vi "Main.vi"(11 "Module Admin":refnum<class "Delacor_lib_QMH_Cloneable Module Admin.lvclass">) -> ()   [LabVIEW 2018, in "CE14 eMIC module.lvlib"]
doc: "This template is based off of the Queued Message Handler design pattern and the Queued Message Handler project template that ships with LabVIEW.\n\nThe main difference is that the queue is private to this module and communication between modules is performed via Broadcast and Request events.\n\nRequest events are wrapped in public API methods and are handled in the Event Handling Loop (EHL) of this VI. Any module can register for Broadcast events sent by this module. The EHL generates messages based on user interface actions.\n\nThe Message Handling Loop (MHL) processes messages generated by the EHL, or by other messages. The messages are string values, so new messages can be added easily to the Message Cases case structure in the MHL. Each message cluster can also provide an optional value for Message Data, which is a variant that can be converted to whatever message-specific data is required.\n_____\nBased on DQMH Project Template 6.0.0.91."
uses:
  CE14 eMIC module.lvlib
  <vilib>/Delacor/Delacor QMH/Libraries/Cloneable Module Admin_class/Delacor_lib_QMH_Cloneable Module Admin.lvclass
  C:/Program Files (x86)/National Instruments/LabVIEW 2018/vi.lib/Delacor/Delacor QMH/Libraries/Module Admin_class/Delacor_lib_QMH_Module Admin.lvclass
  Module Data--cluster.ctl
  Do Something Argument--cluster.ctl
  <vilib>/Delacor/Delacor QMH/Libraries/Cloneable Module Admin_class/Delacor_lib_QMH_Cloneable Module Admin.lvclass/Delacor_lib_QMH_Cloneable Module Admin.ctl
  <vilib>/Delacor/Delacor QMH/Libraries/Message Queue_class/Delacor_lib_QMH_Message Queue.lvclass/Delacor_lib_QMH_Message Queue.ctl
  Do Something Else Argument--cluster.ctl
  Do Something Else and Wait for Reply Argument--cluster.ctl
  Do Something Else and Wait (Reply Payload)--cluster.ctl
  Stop Argument--cluster.ctl
  <vilib>/Delacor/Delacor QMH/Libraries/Module Admin_class/Delacor_lib_QMH_Module Admin.lvclass/Delacor_lib_QMH_Module Admin.ctl
  Open&shakehand eMICs Argument--cluster.ctl
  Open&shakehand eMICs (Reply Payload)--cluster.ctl
  <vilib>/Utility/miscctls.llb/LVPointTypeDef.ctl
  <vilib>/Delacor/Delacor QMH/Libraries/Message Queue_class/Delacor_lib_QMH_Enqueue Message (Single).vi
  <vilib>/Delacor/Delacor QMH/Libraries/Cloneable Module Admin_class/Delacor_lib_QMH_Get Module ID.vi
  <vilib>/Delacor/Delacor QMH/Libraries/Module Admin_class/Delacor_lib_QMH_Get External Launch.vi
  <vilib>/Utility/error.llb/Error Cluster From Error Code.vi
  <vilib>/ErrorRing/Error Ring.xnode
  <vilib>/Delacor/Delacor QMH/Libraries/Message Queue_class/Delacor_lib_QMH_Message Queue.lvclass
  Instrument Drivers/LVdriver_CE14(eMIC)/CE14_eMIC.lvlib
panel:
  out "error out":errorcluster
  out "X":dbl
  out "Status":string
  in  "Simulate EHL Error":bool
  in  "Simulate MHL Error":bool
  in  "Do Something Else <Replace Me>":bool
  in  "Do Something <Replace Me>":bool
  # "These controls have associated \"Value Changed\" events configured in the Event Structure on the diagram.\n\nReplace them (and reconfigure the Event Structure) with the controls you need for your application. \n\nOther QMH Modules communicate with this Module via its Public API (wrappers for its Request Events).\n\nThis Module communicates with other Modules via its Broadcast Events.\nAny module that wants to get these messages, just registers for this module's Broadcast events."
  # "This template is for the Delacor Modified Queued Message Handler design pattern.\n\nSee the block diagram for more information on how to use this template."
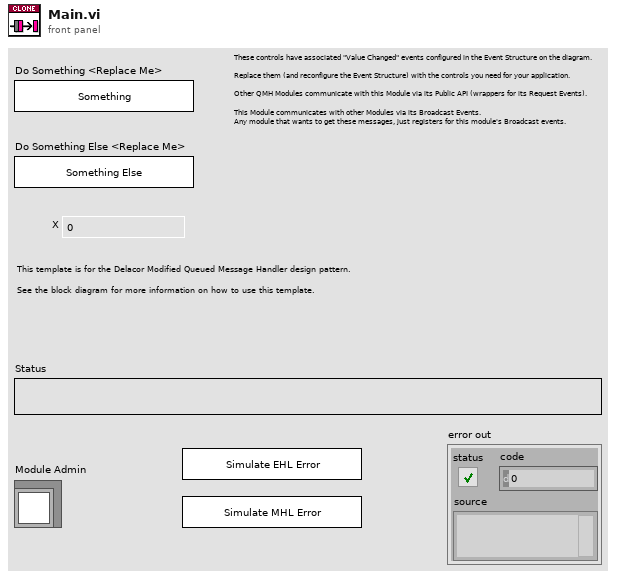
[diagram p1: front panel]
types:
  T1 = typedef "CE14 eMIC module.lvlib/Request Events--cluster.ctl" = cluster{"Stop Module":refnum<user-event>, "Do Something":refnum<user-event>, "Do Something Else":refnum<user-event>, "Do Something Else and Wait for Reply":refnum<user-event>, "Show Panel":refnum<user-event>, "Hide Panel":refnum<user-event>, "Show Diagram":refnum<user-event>, "Get Module Execution Status":refnum<user-event>, "Open&shakehand eMICs":refnum<user-event>}
  T2 = typedef "CE14 eMIC module.lvlib/Module Data--cluster.ctl" = cluster{"Status":string, "VISA resource name":refnum<visa-resource-name>}
  T3 = typedef "CE14 eMIC module.lvlib/Do Something Argument--cluster.ctl" = cluster{"Module ID":i32, "Do Something Msg":string}
  T4 = typedef "CE14 eMIC module.lvlib/Do Something Else Argument--cluster.ctl" = cluster{"Module ID":i32, "Do Something Else Msg":string, "X":dbl}
  T5 = typedef "CE14 eMIC module.lvlib/Do Something Else and Wait for Reply Argument--cluster.ctl" = cluster{"Module ID":i32, "Do Something Else Msg":string, "X":dbl, "Wait Notifier":refnum<notifier>, "wait for reply":bool}
  T6 = enum32{"invalid lock state", "Not Locked", "Locked (No Password)", "Password-protected"}
  T7 = typedef "CE14 eMIC module.lvlib/Stop Argument--cluster.ctl" = cluster{"Module ID":i32, "Origin":string, "Exit via Stop Module Req?":bool, "Wait for Module to stop?":bool}
  T8 = typedef "CE14 eMIC module.lvlib/Open&shakehand eMICs Argument--cluster.ctl" = cluster{"Module ID":i32, "VISA resource name":refnum<visa-resource-name>, "Wait Notifier":refnum<notifier>, "wait for reply":bool}
  T9 = typedef "LVPointTypeDef.ctl" = cluster{"Horizontal":i16, "Vertical":i16}
  T10 = enum32{"Invalid", "Standard", "Closed", "Hidden", "Minimized", "Maximized"}
  T11 = typedef "CE14 eMIC module.lvlib/Do Something Else and Wait (Reply Payload)--cluster.ctl" = cluster{"Value":dbl, "error":errorcluster}
  T12 = typedef "CE14 eMIC module.lvlib/Open&shakehand eMICs (Reply Payload)--cluster.ctl" = cluster{"success":bool, "Open&shakehand eMICs_error":errorcluster}
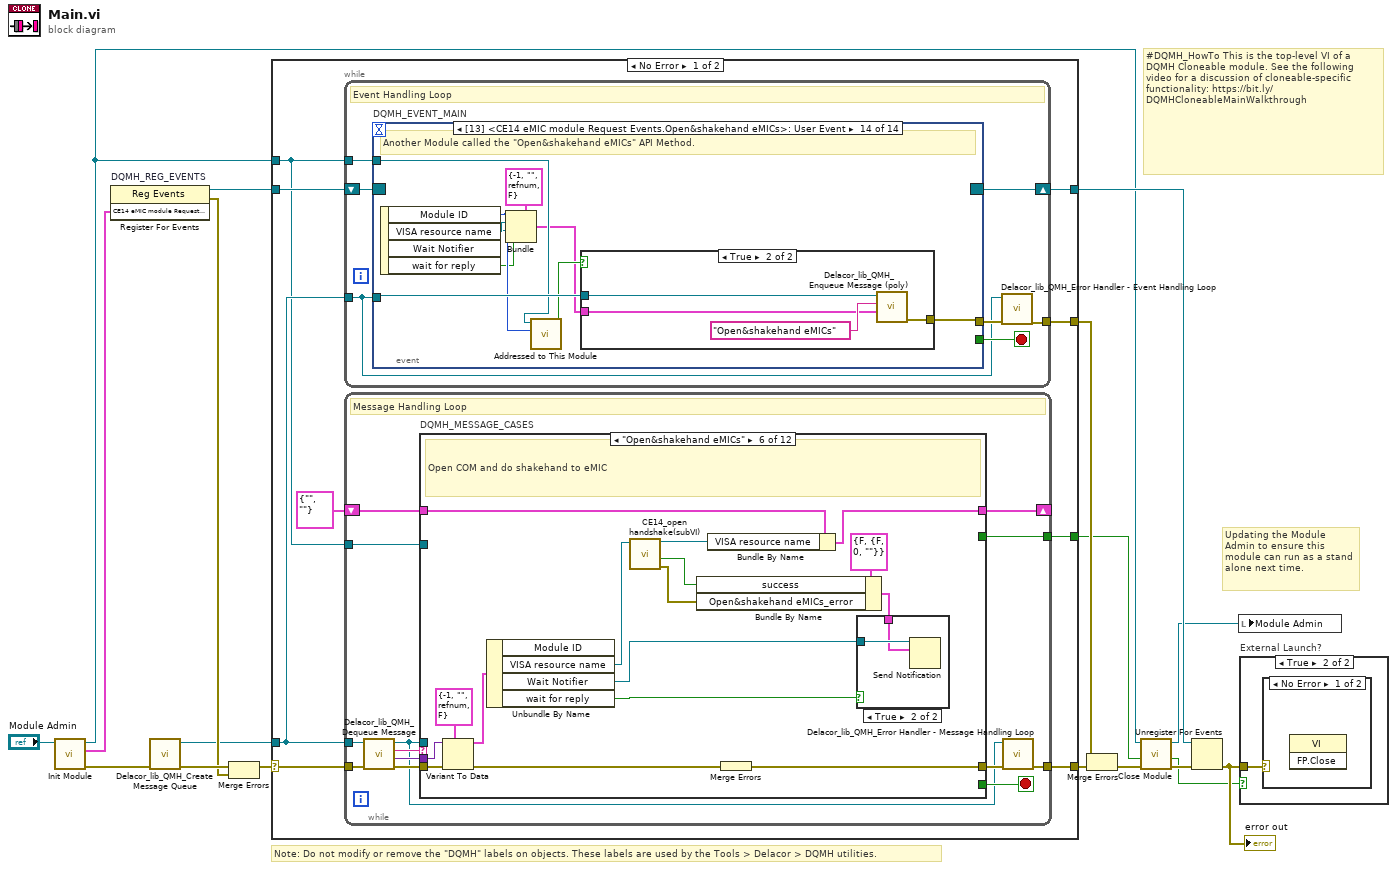
[diagram p0: block diagram]
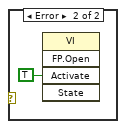
[diagram p3: hidden frame]
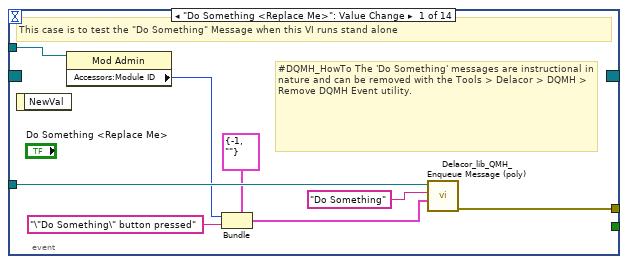
[diagram p4: hidden frame]
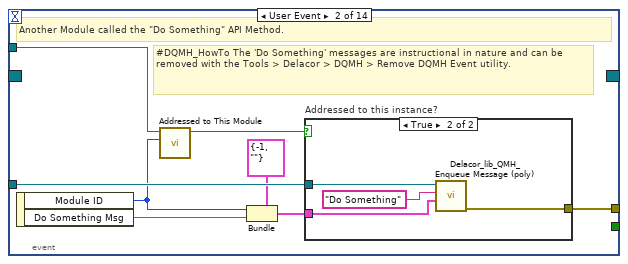
[diagram p5: hidden frame]
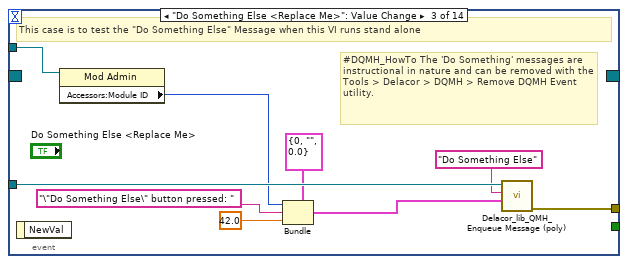
[diagram p7: hidden frame]
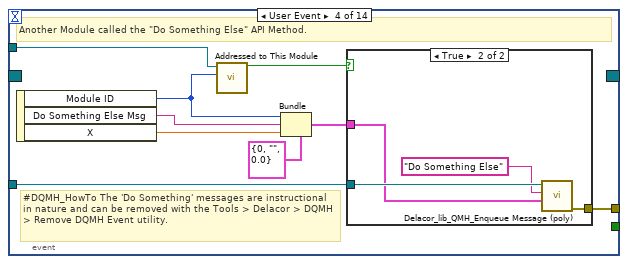
[diagram p8: hidden frame]
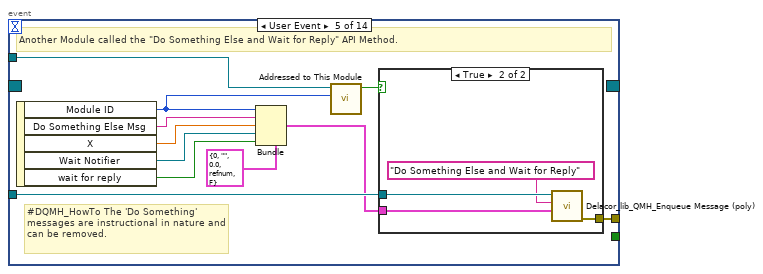
[diagram p10: hidden frame]
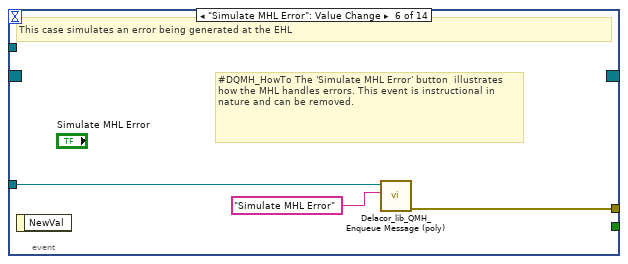
[diagram p12: hidden frame]
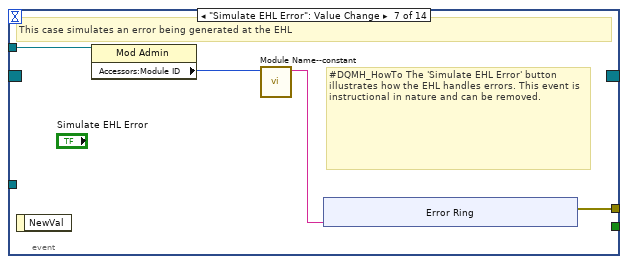
[diagram p13: hidden frame]
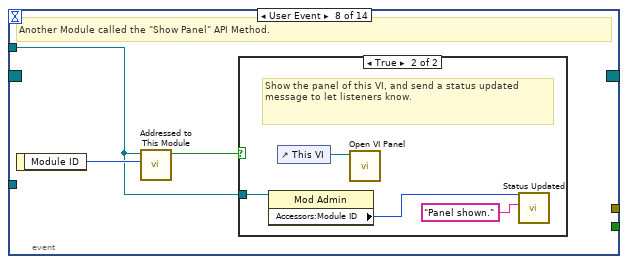
[diagram p14: hidden frame]
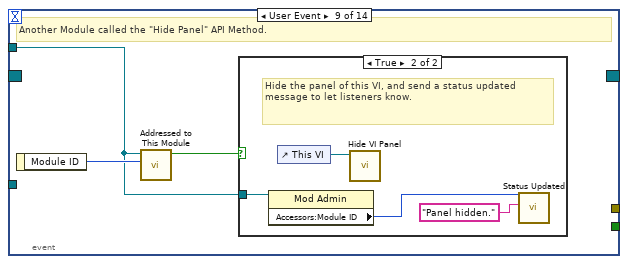
[diagram p16: hidden frame]
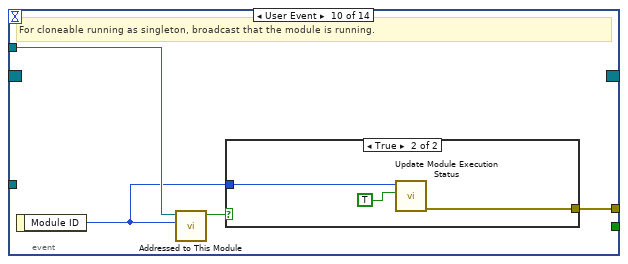
[diagram p18: hidden frame]
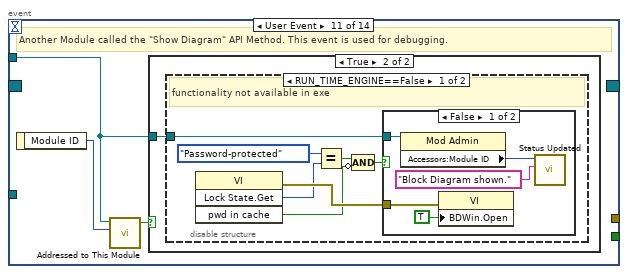
[diagram p20: hidden frame]
diagram:
  # "#DQMH_HowTo This is the top-level VI of a DQMH Cloneable module. See the following video for a discussion of cloneable-specific functionality: https://bit.ly/DQMHCloneableMainWalkthrough"
  # "Note: Do not modify or remove the \"DQMH\" labels on objects. These labels are used by the Tools > Delacor > DQMH utilities."
  # "Updating the Module Admin to ensure this module can run as a stand alone next time."
  n1 = call "Init Module.vi"("Cloneable Module Admin in"="Module Admin") -> ("error out"=w15:errorcluster, "CE14 eMIC module Request Events"=w7:T1, "Cloneable Module Admin out"=w4:refnum<class "Delacor_lib_QMH_Cloneable Module Admin.lvclass">)  [unwired: 8 in]
  n2 = register-events "DQMH_REG_EVENTS"(w7) -> (reference out=w8:refnum<event-registration>, error out=w10:errorcluster)  [unwired: 2 in]
  n3 = call <vilib>:"Delacor_lib_QMH_Create Message Queue.vi"("error in"=w15) -> ("error out"=w12:errorcluster, "Message Queue"=w6:refnum<class "Delacor_lib_QMH_Message Queue.lvclass">)  [unwired: 9 in]
  n4 = Merge Errors(w12, w10) -> (w11:errorcluster)
  n5 = case shown="No Error" w11 {
    selector: w11 -> [w25 w366]
    tunnel: [w27 w365] -> w16
    tunnel: [w24 w373] -> w9
    tunnel: w8 -> [w22 w373]
    tunnel: w6 -> [w21 w364]
    tunnel: [w26 _] -> w17
    tunnel: w4 -> [w20 w369]
    tunnel: [w19 _] -> w2
    frame No Error {
      n6 = while {
        tunnel: w21 -> [w28]
        shift-right: [w31] -> w24
        shift-left: w22 -> [w32]
        tunnel: [w33] -> w26
        tunnel: w20 -> [w29]
        stop <- w30 stop-if-true
        # "Event Handling Loop"
        n7 = event "DQMH_EVENT_MAIN" shown="[13] <CE14 eMIC module Request Events.Open&shakehand eMICs>: User Event" {
          selector: w32 -> [_ _ _ _ _ _ _ _ _ _ _ _ _ _]
          dyn-events: [_ _ _ _ _ _ _ _ _ _ _ _ _ _] -> w31
          timeout: _ -> [_ _ _ _ _ _ _ _ _ _ _ _ _ _]
          tunnel: [_ _ _ _ _ _ _ _ _ _ _ w146 _ _] -> w30
          tunnel: w28 -> [w41 w49 w62 w71 w86 w93 _ _ _ _ _ w149 w165 w183]
          tunnel: [w42 w50 w63 w72 w87 w94 w98 _ _ w123 _ w150 w168 w174] -> w34
          tunnel: w29 -> [w37 w47 w56 w69 w84 _ w97 w106 w113 w121 w127 w148 w166 w181]
          event "Do Something <Replace Me>": Value Change {
            # "#DQMH_HowTo The 'Do Something' messages are instructional in nature and can be removed with the Tools > Delacor > DQMH > Remove DQMH Event utility."
            # "This case is to test the \"Do Something\" Message when this VI runs stand alone"
            n8 = event-data() -> ()  [unwired: 1 in, 1 out]
            n9 = property class="Mod Admin"(reference=w37) -> ("Accessors:Module ID"=w36:i32)  [unwired: 1 in, 2 out]
            n10 = Bundle(cluster=T3 {"Module ID"=-1, "Do Something Msg"=""} ("Do Something Argument"), "Module ID"=w36, "Do Something Msg"="\"Do Something\" button pressed" ("\"Do Something\" button pressed")) -> (w39:T3)
            n11 = call-poly <vilib>:"Delacor_lib_QMH_Enqueue Message (poly).vi"("Message Data"=w39, "Message"="Do Something", "Message Queue in"=w41) -> ("error out"=w42:errorcluster)  [unwired: 7 in, 1 out]
          }
          event User Event {
            # "#DQMH_HowTo The 'Do Something' messages are instructional in nature and can be removed with the Tools > Delacor > DQMH > Remove DQMH Event utility."
            # "Another Module called the \"Do Something\" API Method."
            n12 = event-data() -> ("Module ID"=w44:i32, "Do Something Msg"=w43:string)  [unwired: 1 in]
            n13 = call "Addressed to This Module.vi"("Module ID from Argument"=w44, "Module Admin"=w47) -> ("Addressed to this instance?"=w48:bool)  [unwired: 8 in, 1 out]
            n14 = Bundle(cluster=T3 {"Module ID"=-1, "Do Something Msg"=""} ("Do Something Argument"), "Module ID"=w44, "Do Something Msg"=w43) -> (w46:T3)
            n15 = case "Addressed to this instance?" shown="True" w48 {
              tunnel: w49 -> [_ w53]
              tunnel: [_ w54] -> w50
              tunnel: w46 -> [_ w51]
              frame False {
                # "Do nothing"
              }
              frame True {
                n16 = call-poly <vilib>:"Delacor_lib_QMH_Enqueue Message (poly).vi"("Message Data"=w51, "Message"="Do Something", "Message Queue in"=w53) -> ("error out"=w54:errorcluster)  [unwired: 7 in, 1 out]
              }
            }
          }
          event "Do Something Else <Replace Me>": Value Change {
            # "#DQMH_HowTo The 'Do Something' messages are instructional in nature and can be removed with the Tools > Delacor > DQMH > Remove DQMH Event utility."
            # "This case is to test the \"Do Something Else\" Message when this VI runs stand alone"
            n17 = event-data() -> ()  [unwired: 1 in, 1 out]
            n18 = property class="Mod Admin"(reference=w56) -> ("Accessors:Module ID"=w55:i32)  [unwired: 1 in, 2 out]
            n19 = Bundle(cluster=T4 {"Module ID"=0, "Do Something Else Msg"="", "X"=0.0} ("Do Something Else Argument"), "Module ID"=w55, "Do Something Else Msg"="\"Do Something Else\" button pressed: " ("\"Do Something Else\" button pressed"), "X"=42.0) -> (w59:T4)
            n20 = call-poly <vilib>:"Delacor_lib_QMH_Enqueue Message (poly).vi"("Message Data"=w59, "Message"="Do Something Else", "Message Queue in"=w62) -> ("error out"=w63:errorcluster)  [unwired: 7 in, 1 out]
          }
          event User Event {
            # "#DQMH_HowTo The 'Do Something' messages are instructional in nature and can be removed with the Tools > Delacor > DQMH > Remove DQMH Event utility."
            # "Another Module called the \"Do Something Else\" API Method."
            n21 = event-data() -> ("Module ID"=w64:i32, "Do Something Else Msg"=w65:string, "X"=w67:dbl)  [unwired: 1 in]
            n22 = call "Addressed to This Module.vi"("Module ID from Argument"=w64, "Module Admin"=w69) -> ("Addressed to this instance?"=w70:bool)  [unwired: 8 in, 1 out]
            n23 = Bundle(cluster=T4 {"Module ID"=0, "Do Something Else Msg"="", "X"=0.0} ("Do Something Else Argument"), "Module ID"=w64, "Do Something Else Msg"=w65, "X"=w67) -> (w66:T4)
            n24 = case shown="True" w70 {
              tunnel: w71 -> [_ w75]
              tunnel: [_ w76] -> w72
              tunnel: w66 -> [_ w73]
              frame False {
              }
              frame True {
                n25 = call-poly <vilib>:"Delacor_lib_QMH_Enqueue Message (poly).vi"("Message Data"=w73, "Message"="Do Something Else", "Message Queue in"=w75) -> ("error out"=w76:errorcluster)  [unwired: 7 in, 1 out]
              }
            }
          }
          event User Event {
            # "#DQMH_HowTo The 'Do Something' messages are instructional in nature and can be removed."
            # "Another Module called the \"Do Something Else and Wait for Reply\" API Method."
            n26 = event-data() -> ("Module ID"=w82:i32, "Do Something Else Msg"=w80:string, "X"=w79:dbl, "Wait Notifier"=w78:refnum<notifier>, "wait for reply"=w77:bool)  [unwired: 1 in]
            n27 = Bundle(cluster=T5 {"Module ID"=0, "Do Something Else Msg"="", "X"=0.0, "Wait Notifier"=refnum, "wait for reply"=FALSE} ("Do Something Else and Wait for Reply Argument"), "Module ID"=w82, "Do Something Else Msg"=w80, "X"=w79, "Wait Notifier"=w78, "wait for reply"=w77) -> (w81:T5)
            n28 = call "Addressed to This Module.vi"("Module ID from Argument"=w82, "Module Admin"=w84) -> ("Addressed to this instance?"=w85:bool)  [unwired: 8 in, 1 out]
            n29 = case shown="True" w85 {
              tunnel: [_ w91] -> w87
              tunnel: w86 -> [_ w90]
              tunnel: w81 -> [_ w88]
              frame False {
              }
              frame True {
                n30 = call-poly <vilib>:"Delacor_lib_QMH_Enqueue Message (poly).vi"("Message Data"=w88, "Message"="Do Something Else and Wait for Reply", "Message Queue in"=w90) -> ("error out"=w91:errorcluster)  [unwired: 7 in, 1 out]
              }
            }
          }
          event "Simulate MHL Error": Value Change {
            # "#DQMH_HowTo The 'Simulate MHL Error' button  illustrates how the MHL handles errors. This event is instructional in nature and can be removed."
            # "This case simulates an error being generated at the EHL"
            n31 = event-data() -> ()  [unwired: 1 in, 1 out]
            n32 = call-poly <vilib>:"Delacor_lib_QMH_Enqueue Message (poly).vi"("Message"="Simulate MHL Error", "Message Queue in"=w93) -> ("error out"=w94:errorcluster)  [unwired: 8 in, 1 out]
          }
          event "Simulate EHL Error": Value Change {
            # "#DQMH_HowTo The 'Simulate EHL Error' button  illustrates how the EHL handles errors. This event is instructional in nature and can be removed."
            # "This case simulates an error being generated at the EHL"
            n33 = event-data() -> ()  [unwired: 1 in, 1 out]
            n34 = property class="Mod Admin"(reference=w97) -> ("Accessors:Module ID"=w96:i32)  [unwired: 1 in, 2 out]
            n35 = call "Module Name--constant.vi"("Module ID"=w96) -> ("Module Name"=w95:string)  [unwired: 10 in]
            n36 = xnode "Error Ring"("parameter 0"=w95) -> ("error out"=w98:errorcluster)
          }
          event User Event {
            # "Another Module called the \"Show Panel\" API Method."
            n37 = event-data() -> ("Module ID"=w107:i32)  [unwired: 1 in]
            n38 = call "Addressed to This Module.vi"("Module ID from Argument"=w107, "Module Admin"=w106) -> ("Addressed to this instance?"=w108:bool)  [unwired: 8 in, 1 out]
            n39 = case shown="True" w108 {
              tunnel: w106 -> [_ w110]
              frame False {
              }
              frame True {
                # "Show the panel of this VI, and send a status updated message to let listeners know."
                n40 = property class="Mod Admin"(reference=w110) -> ("Accessors:Module ID"=w109:i32)  [unwired: 1 in, 2 out]
                n41 = control-ref of="This VI"() -> (w112:refnum<vi>)
                n42 = call "Open VI Panel.vi"("VI"=w112) -> ()  [unwired: 10 in, 1 out]
                n43 = call "Status Updated.vi"("Status"="Panel shown." ("format string"), "Module ID"=w109) -> ()  [unwired: 9 in, 1 out]
              }
            }
          }
          event User Event {
            # "Another Module called the \"Hide Panel\" API Method."
            n44 = event-data() -> ("Module ID"=w114:i32)  [unwired: 1 in]
            n45 = call "Addressed to This Module.vi"("Module ID from Argument"=w114, "Module Admin"=w113) -> ("Addressed to this instance?"=w115:bool)  [unwired: 8 in, 1 out]
            n46 = case shown="True" w115 {
              tunnel: w113 -> [_ w117]
              frame False {
              }
              frame True {
                # "Hide the panel of this VI, and send a status updated message to let listeners know."
                n47 = property class="Mod Admin"(reference=w117) -> ("Accessors:Module ID"=w116:i32)  [unwired: 1 in, 2 out]
                n48 = control-ref of="This VI"() -> (w119:refnum<vi>)
                n49 = call "Hide VI Panel.vi"("VI"=w119) -> ()  [unwired: 10 in, 1 out]
                n50 = call "Status Updated.vi"("Status"="Panel hidden." ("format string"), "Module ID"=w116) -> ()  [unwired: 9 in, 1 out]
              }
            }
          }
          event User Event {
            # "For cloneable running as singleton, broadcast that the module is running."
            n51 = event-data() -> ("Module ID"=w120:i32)  [unwired: 1 in]
            n52 = call "Addressed to This Module.vi"("Module ID from Argument"=w120, "Module Admin"=w121) -> ("Addressed to this instance?"=w122:bool)  [unwired: 8 in, 1 out]
            n53 = case shown="True" w122 {
              tunnel: [_ w126] -> w123
              tunnel: w120 -> [_ w125]
              frame False {
              }
              frame True {
                n54 = call "Update Module Execution Status.vi"("Running?"=TRUE, "Module ID"=w125) -> ("error out"=w126:errorcluster)  [unwired: 9 in]
              }
            }
          }
          event User Event {
            # "Another Module called the \"Show Diagram\" API Method. This event is used for debugging."
            n55 = event-data() -> ("Module ID"=w128:i32)  [unwired: 1 in]
            n56 = call "Addressed to This Module.vi"("Module ID from Argument"=w128, "Module Admin"=w127) -> ("Addressed to this instance?"=w129:bool)  [unwired: 8 in, 1 out]
            n57 = case shown="True" w129 {
              tunnel: w127 -> [_ w130]
              frame False {
              }
              frame True {
                n58 = disable-structure shown="RUN_TIME_ENGINE==False" {
                  disable-tunnel: w130 -> [w131 _]
                  frame condition #0 (active) {
                    # "functionality not available in exe"
                    n59 = invoke class="VI" method="Lock State.Get"() -> (error out=w137:errorcluster, "Get Lock State"=w136:T6, "pwd in cache"=w133:bool)  [unwired: 4 in, 1 out]
                    n60 = Equal?(x=T6."Password-protected", y=w136) -> (x = y?=w134:bool)
                    n61 = Compound Arithmetic op=AND(w134, invert w133) -> (w132:bool)
                    n62 = case shown="False" w132 {
                      tunnel: w137 -> [w142 _]
                      tunnel: w131 -> [w139 _]
                      frame False {
                        n63 = property class="Mod Admin"(reference=w139) -> ("Accessors:Module ID"=w138:i32)  [unwired: 1 in, 2 out]
                        n64 = property class="VI"(error in=w142, "BDWin.Open"=TRUE ("Block Diagram Window:Open")) -> ()  [unwired: 1 in, 2 out]
                        n65 = call "Status Updated.vi"("Status"="Block Diagram shown." ("format string"), "Module ID"=w138) -> ()  [unwired: 9 in, 1 out]
                      }
                      frame True {
                        # "Password-protected VI, and the password is not in the cache. Do not show the diagram."
                      }
                    }
                  }
                  frame condition #1 {
                  }
                }
              }
            }
          }
          event User Event {
            # "Another Module called the \"Stop Module\" API Method  or the Message Handling Loop below."
            n66 = event-data() -> ("Module ID"=w144:i32, "Wait for Module to stop?"=w145:bool, "Origin"=w143:string)  [unwired: 1 in]
            n67 = call "Addressed to This Module.vi"("Module ID from Argument"=w144, "Module Admin"=w148) -> ("Addressed to this instance?"=w147:bool)  [unwired: 8 in, 1 out]
            n68 = case shown="True" w147 {
              tunnel: [_ w162] -> w150
              tunnel: w149 -> [_ w158]
              tunnel: [_ TRUE] -> w146
              tunnel: w145 -> [_ w153]
              tunnel: w144 -> [_ w155]
              tunnel: w143 -> [_ w151]
              frame False {
              }
              frame True {
                # "The event can get fired from the Exit message. The queue gets destroyed there. In this case, the Enqueue VI will return error 1. It is safe to ignore, because the module is already exiting."
                n69 = local write "Status"(w151) -> ()
                n70 = Bundle By Name(cluster=T7 {"Module ID"=-1, "Origin"="", "Exit via Stop Module Req?"=FALSE, "Wait for Module to stop?"=FALSE} ("Stop Argument"), "Module ID"=w155, "Exit via Stop Module Req?"=TRUE, "Wait for Module to stop?"=w153) -> (w152:T7)
                n71 = call-poly <vilib>:"Delacor_lib_QMH_Enqueue Message (poly).vi"("Priority Message? (F)"=TRUE, "Message Data"=w152, "Message"="Exit", "Message Queue in"=w158) -> ("error out"=w163:errorcluster)  [unwired: 6 in, 1 out]
                n72 = call <vilib>:"Clear Errors.vi"("error in (no error)"=w163, "specific error code to clear (0: all)"=1) -> ("error out"=w162:errorcluster)  [unwired: 4 in, 1 out]
              }
            }
          }
          event Panel Close? {
            w167 = TRUE  # Discard the event, the MHL is responsible for closing and stopping this VI.
            # "Hide the panel or send the 'Exit' message if the user clicks the 'X' on the module main VI panel."
            n73 = event-data() -> ()  [unwired: 1 in, 1 out]
            n74 = property class="Mod Admin"(reference=w166) -> ("Accessors:External Launch"=w164:bool)  [unwired: 1 in, 2 out]
            n75 = case shown="True" w164 {
              tunnel: w165 -> [_ w172]
              tunnel: [_ w173] -> w168
              frame True {
                # "If externally launched, clicking the 'X' hides the panel, but doesn't close it."
                n76 = control-ref of="This VI"() -> (w169:refnum<vi>)
                n77 = call "Hide VI Panel.vi"("VI"=w169) -> ()  [unwired: 10 in, 1 out]
              }
              frame False {
                # "If run as a stand-alone VI, clicking the panel 'X' stops the VI."
                n78 = call-poly <vilib>:"Delacor_lib_QMH_Enqueue Message (poly).vi"("Priority Message? (F)"=TRUE, "Message"="Exit", "Message Queue in"=w172) -> ("error out"=w173:errorcluster)  [unwired: 7 in, 1 out]
              }
            }
            n79 = event-data("Discard?"=w167) -> ()  [unwired: 1 in, 1 out]
          }
          event User Event {
            # "Another Module called the \"Open&shakehand eMICs\" API Method."
            n80 = event-data() -> ("Module ID"=w178:i32, "VISA resource name"=w177:refnum<visa-resource-name>, "Wait Notifier"=w176:refnum<notifier>, "wait for reply"=w175:bool)  [unwired: 1 in]
            n81 = Bundle(cluster=T8 {"Module ID"=-1, "VISA resource name"="", "Wait Notifier"=refnum, "wait for reply"=FALSE} ("Open&shakehand eMICs Argument"), "Module ID"=w178, "VISA resource name"=w177, "Wait Notifier"=w176, "wait for reply"=w175) -> (w179:T8)
            n82 = call "Addressed to This Module.vi"("Module ID from Argument"=w178, "Module Admin"=w181) -> ("Addressed to this instance?"=w182:bool)  [unwired: 8 in, 1 out]
            n83 = case shown="True" w182 {
              tunnel: w183 -> [_ w187]
              tunnel: w179 -> [_ w185]
              tunnel: [_ w184] -> w174
              frame False {
              }
              frame True {
                n84 = call-poly <vilib>:"Delacor_lib_QMH_Enqueue Message (poly).vi"("Message Data"=w185, "Message"="Open&shakehand eMICs", "Message Queue in"=w187) -> ("error out"=w184:errorcluster)  [unwired: 7 in, 1 out]
              }
            }
          }
        }
        n85 = call-dynamic "Delacor_lib_QMH_Error Handler - Event Handling Loop.vi"("error in"=w34, "Message Queue in"=w28) -> ("dup error in"=w33:errorcluster)  [unwired: 8 in, 1 out]
      }
      n86 = while {
        tunnel: w21 -> [w191]
        shift-right: [w195] -> _
        shift-left: T2 {"Status"="", "VISA resource name"=""} ("Data Cluster") -> [w196]
        tunnel: w25 -> [w199]
        tunnel: [w197] -> w27
        tunnel: w20 -> [w189]
        tunnel: [w188] -> w19
        stop <- w194 stop-if-true
        # "Message Handling Loop"
        n87 = call-dynamic "Delacor_lib_QMH_Dequeue Message.vi"("error in"=w199, "Message Queue in"=w191) -> ("error out"=w198:errorcluster, "Message Data"=w192:variant, "Message"=w193:string, "Message Queue out"=w190:refnum<class "Delacor_lib_QMH_Message Queue.lvclass">)  [unwired: 6 in]
        n88 = case "DQMH_MESSAGE_CASES" shown="\"Open&shakehand eMICs\"" w193 {
          selector: w193 -> [_ _ _ _ _ _ _ _ _ _ _ w351]
          tunnel: w190 -> [_ _ _ _ _ _ _ _ w302 _ w341 _]
          tunnel: w198 -> [w219 w223 w233 w244 w265 w293 w298 w300 w311 w324 w347 w353]
          tunnel: [w217 w223 w231 w243 w264 w284 w297 w300 w307 w323 w344 w354] -> w200
          tunnel: w196 -> [w210 w222 w230 w242 w262 w279 w296 w299 w306 w321 w340 w352]
          tunnel: [w209 w222 w230 w242 w262 w280 w296 w299 w306 w321 w340 w352] -> w195
          tunnel: [_ _ _ _ _ _ _ _ _ _ w339 _] -> w194
          tunnel: w192 -> [_ _ w229 w239 w259 w291 _ _ w305 _ w337 _]
          tunnel: w189 -> [w204 _ w225 w235 w249 _ _ _ w304 w319 w333 w349]
          tunnel: [_ _ _ _ _ _ _ _ _ _ w335 _] -> w188
          frame "Initialize" {
            w201 = "Initial Message" ("Initial Message")
            # "#CodeNeeded - Initialize the appearance of the front panel."
            # "#CodeNeeded - Initialize your state data here."
            # "Initialize - Any operation that needs to be done before the module can receive messages. Synchronize Caller Events.vi will inform Start Module.vi that the module has launched and is ready to receive messages. Module Did Init.vi will broadcast that the module initialized."
            n89 = call "Synchronize Caller Events.vi"("error in (no error)"=w219, "Module Admin"=w204) -> ("error out"=w218:errorcluster, "Module Admin out"=w203:refnum<class "Delacor_lib_QMH_Cloneable Module Admin.lvclass">)  [unwired: 8 in]
            n90 = property class="Mod Admin"(reference=w203) -> ("Accessors:Module ID"=w206:i32, "Accessors:External Launch"=w205:bool)  [unwired: 1 in, 2 out]
            n91 = call "Module Name--constant.vi"("Module ID"=w206) -> ("Module Name"=w214:string)  [unwired: 10 in]
            n92 = property class="VI"("Front Panel.Title"=w214) -> (reference out=w216:refnum<vi>, error out=w221:errorcluster)  [unwired: 2 in]
            n93 = Select(t=T10."Hidden" ("State"), s=w205, f=T10."Standard" ("State")) -> (s? t:f=w211:T10)
            n94 = invoke class="VI" method="FP.Open"(reference=w216, error in=w221, "State"=w211) -> (reference out=w215:refnum<vi>, error out=w220:errorcluster)  [unwired: 2 in, 3 out]
            n95 = call "Module Name--constant.vi"("Module ID"=w206) -> ("Module Name"=w207:string)  [unwired: 10 in]
            n96 = Bundle By Name(cluster=w210, "Status"=w201) -> (w209:T2)
            n97 = invoke class="VI" method="FP.Center"(reference=w215, error in=w220) -> ()  [unwired: 1 in, 3 out]
            n98 = property on="Pane" class="Pane"("Origin"=T9 {"Horizontal"=0, "Vertical"=0}) -> ()  [unwired: 2 in, 2 out]
            n99 = call "Module Did Init.vi"("error in (no error)"=w218, "Initialized?"=TRUE, "Origin"=w207, "Module ID"=w206) -> ("error out"=w217:errorcluster)  [unwired: 7 in]
            "Status" <- w201
          }
          frame "---Module Specific---" {
            # "Separator -- The following cases handle messages specific to this Module."
          }
          frame "Do Something" {
            # "#DQMH_HowTo The 'Do Something' messages are instructional in nature and can be removed with the Tools > Delacor > DQMH > Remove DQMH Event utility."
            # "Do Something - Replace this message with functionality for your own application. Note that this message also fires the \"Did Something\" broadcast event."
            n100 = property class="Mod Admin"(reference=w225) -> ("Accessors:Module ID"=w224:i32)  [unwired: 1 in, 2 out]
            n101 = Variant To Data(error in=w233, type=T3 {"Module ID"=-1, "Do Something Msg"=""} ("Do Something Argument"), Variant=w229) -> (data=w228:T3, error out=w232:errorcluster)
            n102 = Unbundle By Name(w228) -> ("Do Something Msg"=w226:string)
            n103 = call "Status Updated.vi"("Status"=w226, "Module ID"=w224) -> ()  [unwired: 9 in, 1 out]
            n104 = local write "Status"(w226) -> ()
            n105 = call "Did Something.vi"("error in (no error)"=w232, "Did Something Msg"=w226, "Module ID"=w224) -> ("error out"=w231:errorcluster)  [unwired: 8 in]
          }
          frame "Do Something Else" {
            # "#DQMH_HowTo The 'Do Something' messages are instructional in nature and can be removed with the Tools > Delacor > DQMH > Remove DQMH Event utility."
            # "Do Something Else - Replace this message with functionality for your own application."
            n106 = Variant To Data(error in=w244, type=T4 {"Module ID"=0, "Do Something Else Msg"="", "X"=0.0} ("Do Something Else Argument"), Variant=w239) -> (data=w240:T4, error out=w243:errorcluster)
            n107 = Unbundle By Name(w240) -> ("Do Something Else Msg"=w238:string, "X"=w237:dbl)
            "X" <- w237
            n108 = property class="Mod Admin"(reference=w235) -> ("Accessors:Module ID"=w234:i32)  [unwired: 1 in, 2 out]
            n109 = Format Into String(initial string=w238, w237) -> (resulting string=w236:string)  [unwired: 2 in, 1 out]
            n110 = call "Status Updated.vi"("Status"=w236, "Module ID"=w234) -> ()  [unwired: 9 in, 1 out]
            n111 = local write "Status"(w236) -> ()
          }
          frame "Do Something Else and Wait for Reply" {
            w252 = "X(%.2f)+Offset(%.2f)=%.2f"  # status message format string
            # "#DQMH_HowTo The 'Do Something' messages are instructional in nature and can be removed."
            # "Send back X with a random offset"
            # "Do Something Else and Wait for Reply - Replace this message with functionality for your own application. Note that this message must fire a notifier to let callers know it has finished execution, and it returns an error if the 'Value' is negative."
            n112 = Variant To Data(error in=w265, type=T5 {"Module ID"=0, "Do Something Else Msg"="", "X"=0.0, "Wait Notifier"=refnum, "wait for reply"=FALSE} ("Do Something Else and Wait for Reply Argument"), Variant=w259) -> (data=w260:T5, error out=w246:errorcluster)
            n113 = Unbundle By Name(w260) -> ("Wait Notifier"=w257:refnum<notifier>, "Do Something Else Msg"=w258:string, "X"=w254:dbl, "wait for reply"=w245:bool)
            n114 = property class="Mod Admin"(reference=w249) -> ("Accessors:Module ID"=w248:i32)  [unwired: 1 in, 2 out]
            n115 = Random Number (0-1)() -> (number: 0 to 1=w253:dbl)
            n116 = local write "X"(w254) -> ()
            n117 = Add(x=w253, y=w254) -> (x+y=w247:dbl)
            n118 = Format Into String(format string=w252, initial string=w258, w254, w253, w247) -> (resulting string=w250:string)  [unwired: 1 in, 1 out]
            n119 = Less Than 0?(x=w247) -> (x < 0?=w251:bool)
            n120 = case shown="True" w251 {
              tunnel: [_ w272] -> w263
              frame False {
              }
              frame True {
                n121 = xnode "Error Ring"() -> ("error out"=w272:errorcluster)
              }
            }
            n122 = Bundle By Name(cluster=T11 {"Value"=0.0, "error"={"status"=FALSE, "code"=0, "source"=""}} ("notification"), "error"=w263, "Value"=w247) -> (w255:T11)
            n123 = local write "Status"(w250) -> ()
            n124 = call "Status Updated.vi"("Status"=w250, "Module ID"=w248) -> ()  [unwired: 9 in, 1 out]
            n125 = case shown="True" w245 {
              tunnel: w257 -> [_ w269]
              tunnel: w255 -> [_ w268]
              frame False {
              }
              frame True {
                # "Simulate an operation that requires a wait."
                n126 = Wait (ms)(milliseconds to wait=u32 1000) -> (millisecond timer value=w266:u32)
                n127 = flat-sequence {
                  tunnel: w269 -> [w271]
                  tunnel: w268 -> [w270]
                  tunnel: w266 -> [_]
                  frame #0 {
                    n128 = Send Notification(notification=w270, notifier=w271) -> ()  [unwired: 1 in, 2 out]
                  }
                }
              }
            }
            n129 = Merge Errors(w246, w263) -> (w264:errorcluster)
          }
          frame "Open&shakehand eMICs" {
            # "Open COM and do shakehand to eMIC"
            n130 = Variant To Data(error in=w293, type=T8 {"Module ID"=-1, "VISA resource name"="", "Wait Notifier"=refnum, "wait for reply"=FALSE} ("Open&shakehand eMICs Argument"), Variant=w291) -> (data=w289:T8, error out=w292:errorcluster)
            n131 = Unbundle By Name(w289) -> ("VISA resource name"=w282:refnum<visa-resource-name>, "Wait Notifier"=w288:refnum<notifier>, "wait for reply"=w287:bool)  [unwired: 1 out]
            n132 = call "CE14_open handshake(subVI).vi"("VISA resource name"=w282) -> ("error out"=w278:errorcluster, "success"=w283:bool, "VISA resource name 2"=w281:refnum<visa-resource-name>)  [unwired: 7 in, 1 out]
            n133 = Bundle By Name(cluster=T12 {"success"=FALSE, "Open&shakehand eMICs_error"={"status"=FALSE, "code"=0, "source"=""}} ("Open&shakehand eMICs (Reply Payload)"), "success"=w283, "Open&shakehand eMICs_error"=w278) -> (w286:T12)
            n134 = Bundle By Name(cluster=w279, "VISA resource name"=w281) -> (w280:T2)
            n135 = Merge Errors(w292) -> (w284:errorcluster)
            n136 = case shown="True" w287 {
              tunnel: w288 -> [_ w295]
              tunnel: w286 -> [_ w294]
              frame False {
              }
              frame True {
                n137 = Send Notification(notification=w294, notifier=w295) -> ()  [unwired: 1 in, 2 out]
              }
            }
          }
          frame "---Copy This Frame---" {
            # "Duplicate this frame when creating new messages.  Change this comment in the duplicated frame to describe this message."
            n138 = Merge Errors(w298) -> (w297:errorcluster)
          }
          frame "---Exit and Error Handling---" {
            # "Separator - the following cases handle errors and exit messages."
          }
          frame "Error" {
            # "#CodeRecommended - If you ever change the name of this \"Error\" message, you'll need to update the name in the Check Loop Error.vi as well."
            # "#CodeRecommended - If the module is running in standalone mode (External Launch = FALSE), this code will pop up an error dialog and call the 'Exit' message if an error occurs. Add more fine-grained error handling here."
            # "Error - Check the error message data and respond accordingly. This message is sent by the \"Error Handler\" VIs at the end of each loop in this application."
            n139 = property class="Mod Admin"(reference=w304) -> ("Accessors:External Launch"=w303:bool, "Accessors:Module ID"=w301:i32)  [unwired: 1 in, 2 out]
            n140 = Variant To Data(error in=w311, type=errorcluster {"status"=FALSE, "code"=0, "source"=""} ("error constant"), Variant=w305) -> (data=w312:errorcluster, error out=w309:errorcluster)
            n141 = call "Error Reported.vi"("Error"=w312, "Module ID"=w301) -> ()  [unwired: 9 in, 1 out]
            n142 = case shown="False" w303 {
              tunnel: [w317 _] -> w308
              tunnel: w302 -> [w315 _]
              tunnel: w312 -> [w316 _]
              frame False {
                # "If the module is running standalone, then pop up an error dialog and call the \"Exit\" message."
                n143 = call <vilib>:"Simple Error Handler.vi"("error in (no error)"=w316) -> ()  [unwired: 4 in, 5 out]
                n144 = call-poly <vilib>:"Delacor_lib_QMH_Enqueue Message (poly).vi"("Priority Message? (F)"=TRUE, "Message"="Exit", "Message Queue in"=w315) -> ("error out"=w317:errorcluster)  [unwired: 7 in, 1 out]
              }
              frame True {
                # "If the module was launched externally, calling the Error Reported broadcast VI is the only action performed by the \"Error\" message. The module's caller can then process the error appropriately."
              }
            }
            n145 = Merge Errors(w309, w308) -> (w307:errorcluster)
            n146 = local write "error out"(w307) -> ()
          }
          frame "Simulate MHL Error" {
            # "#DQMH_HowTo The 'Simulate MHL Error' button  illustrates how the MHL handles errors. This event is instructional in nature and can be removed."
            # "Simulate an error occurring at the MHL"
            n147 = property class="Mod Admin"(reference=w319) -> ("Accessors:Module ID"=w320:i32)  [unwired: 1 in, 2 out]
            n148 = call "Module Name--constant.vi"("Module ID"=w320) -> ("Module Name"=w318:string)  [unwired: 10 in]
            n149 = xnode "Error Ring"("parameter 0"=w318) -> ("error out"=w322:errorcluster)
            n150 = Merge Errors(w324, w322) -> (w323:errorcluster)
          }
          frame "Exit" {
            w338 = 91  # 91: not all Exit messages will have an argument
            w339 = TRUE  # Stop the VI
            # "Release the message queue reference"
            # "#CodeNeeded - Add any required cleanup code here."
            # "Exit - Exit the application."
            n151 = Variant To Data(error in=w347, type=T7 {"Module ID"=-1, "Origin"="", "Exit via Stop Module Req?"=FALSE, "Wait for Module to stop?"=FALSE} ("Stop Argument"), Variant=w337) -> (data=w334:T7, error out=w342:errorcluster)
            n152 = call <vilib>:"Clear Errors.vi"("error in (no error)"=w342, "specific error code to clear (0: all)"=w338) -> ("error out"=w346:errorcluster)  [unwired: 4 in, 1 out]
            n153 = control-ref of="This VI"() -> (w332:refnum<vi>)
            n154 = call-dynamic "Delacor_lib_QMH_Release Message Queue.vi"("error in"=w346, "Message Queue"=w341) -> ("error out"=w345:errorcluster)  [unwired: 9 in]
            n155 = call "Handle Exit.vi"("Stop Argument"=w334, "Module Admin in"=w333, "VI reference"=w332) -> ("error out"=w343:errorcluster, "Wait for Stop?"=w335:bool)  [unwired: 7 in]
            n156 = Merge Errors(w345, w343) -> (w344:errorcluster)
          }
          frame Default {
            # "'Default' case only runs if there is a message that isn't defined in any of the other cases.  Output a programming error."
            n157 = property class="Mod Admin"(reference=w349) -> ("Accessors:Module ID"=w348:i32)  [unwired: 1 in, 2 out]
            n158 = call "Module Name--constant.vi"("Module ID"=w348) -> ("Module Name"=w350:string)  [unwired: 10 in]
            n159 = xnode "Error Ring"("parameter 0"=w351, "parameter 1"=w350) -> ("error out"=w355:errorcluster)
            n160 = Merge Errors(w353, w355) -> (w354:errorcluster)
          }
        }
        n161 = call-dynamic "Delacor_lib_QMH_Error Handler - Message Handling Loop.vi"("error in"=w200, "Message Queue in"=w190) -> ("dup error in"=w197:errorcluster)  [unwired: 8 in, 1 out]
      }
    }
    frame Error {
      n162 = call "Synchronize Caller Events.vi"("Module Admin"=w369) -> ("Module Admin out"=w368:refnum<class "Delacor_lib_QMH_Cloneable Module Admin.lvclass">)  [unwired: 9 in, 1 out]
      n163 = property class="Mod Admin"(reference=w368) -> ("Accessors:Module ID"=w367:i32)  [unwired: 1 in, 2 out]
      n164 = call-dynamic "Delacor_lib_QMH_Release Message Queue.vi"("error in"=w366, "Message Queue"=w364) -> ("error out"=w365:errorcluster)  [unwired: 9 in]
      n165 = call "Module Name--constant.vi"("Module ID"=w367) -> ("Module Name"=w372:string)  [unwired: 10 in]
      n166 = Format Into String(format string="An error occurred during initialization. %s is no longer running.", w372) -> (resulting string=w370:string)  [unwired: 2 in, 1 out]
      n167 = call "Error Reported.vi"("Additional Information"=w370, "Error"=w365, "Module ID"=w367) -> ()  [unwired: 8 in, 1 out]
    }
  }
  n168 = Merge Errors(w17, w16) -> (w18:errorcluster)
  n169 = call "Close Module.vi"("error in"=w18, "Wait for stop?"=w2, "Module Admin in"=w4) -> ("error out"=w14:errorcluster, "External Launch"=w1:bool, "Module Admin out"=w3:refnum<class "Delacor_lib_QMH_Cloneable Module Admin.lvclass">)  [unwired: 6 in]
  n170 = Unregister For Events(event registration refnum=w9, error in=w14) -> (error out=w13:errorcluster)
  "error out" <- w13
  n171 = local write "Module Admin"(w3) -> ()
  n172 = case "External Launch?" shown="True" w1 {
    tunnel: w13 -> [_ w374]
    frame False {
    }
    frame True {
      n173 = case shown="No Error" w374 {
        frame No Error {
          n174 = invoke class="VI" method="FP.Close"() -> ()  [unwired: 3 in, 3 out]
        }
        frame Error {
          n175 = invoke class="VI" method="FP.Open"("Activate"=TRUE ("Activate?")) -> ()  [unwired: 4 in, 5 out]
        }
      }
    }
  }
